vi "Write Model.vi"(8 "error in":errorcluster, 10 "Model":string, 11 "Base Software in":refnum<class "Base Software.lvclass">) -> (0 "error out":errorcluster, 3 "Base Software out":refnum<class "Base Software.lvclass">)   [LabVIEW 2019, in "Base Software.lvlib" / "Main.lvlib" / "Base Software.lvclass"]
uses:
  Project/Base Software.lvclass
  Project/Base Software.lvclass/Base Software.ctl
  Custom Controls/Color_Items.ctl
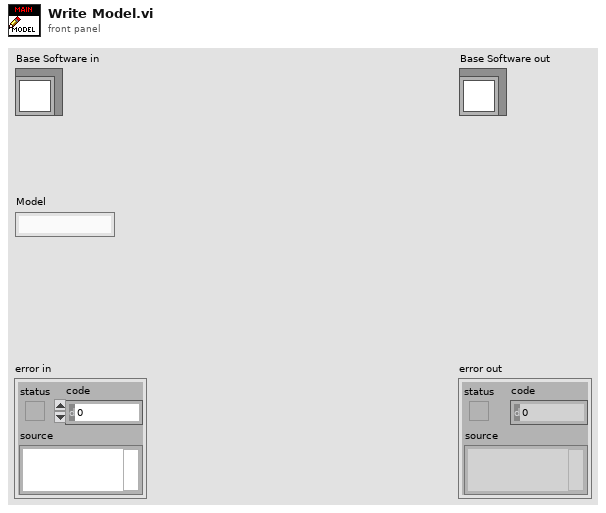
[diagram p1: front panel]
types:
  T1 = typedef "Base Software.lvlib/Main.lvlib/Base Software.lvclass/Color_Items.ctl" = enum16{"Nominal_Low_Impact", "Nominal", "User_Interaction", "Warning", "Error"}
  T2 = typedef "LVTextColorsTypeDef.ctl" = cluster{"Text Color":u32, "Background Color":u32}
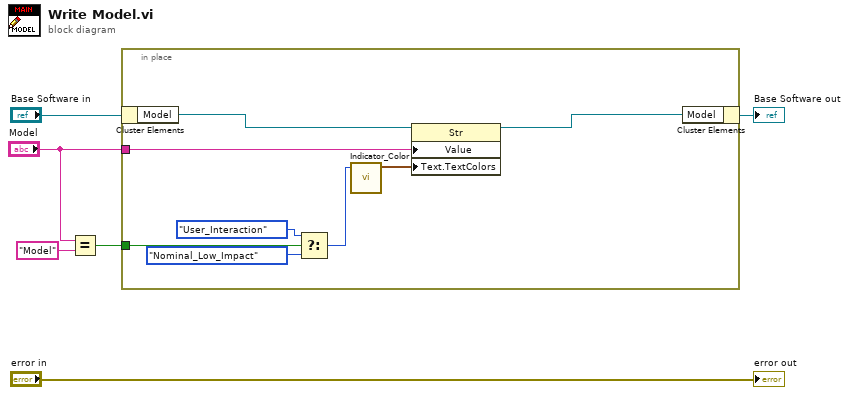
[diagram p0: block diagram]
diagram:
  n1 = Equal?(x="Model", y="Model") -> (x = y?=w1:bool)
  n2 = in-place {
    in-place-border: "Model" -> [w13]
    in-place-border: w1 -> [w11]
    n3 = in-place-cluster #1("Base Software in") -> ("Model"=w8:refnum<vi>)
    n4 = Select(t=Color_Items."User_Interaction" ("Color Selector"), s=w11, f=Color_Items."Nominal_Low_Impact" ("Color Selector")) -> (s? t:f=w9:T1)
    n5 = call "Indicator_Color.vi"("Color Selector"=w9) -> ("Text Colors"=w14:T2)  [unwired: 10 in]
    n6 = property class="Str"(reference=w8, "Value"=w13, "Text.TextColors"=w14) -> (reference out=w7:refnum<vi>)  [unwired: 1 in, 1 out]
    n7 = in-place-cluster #1("Model"=w7) -> (→"Base Software out":refnum<class "Base Software.lvclass">)
  }
  "error out" <- "error in"
